vi "Project_GUI.vi"() -> ()   [LabVIEW 2026]
uses:
  <vilib>/Instr/_visa.llb/VISA Configure Serial Port (Instr).vi
panel:
  in  "Display ON/OFF":bool
  in  "stop":bool
  out "Last Command Sent":string
  out "ESP Response":string
  in  "Send Filters":bool
  in  "Detection Threshold":dbl(knob) scale=0.0..255.0
  in  "Blur":dbl(knob) scale=0.0..10.0
  in  "Minimum Area":dbl
  in  "Get Status":bool
  in  "Reset Filters":bool
  in  "Identify":bool
  out "Connected to ESP":bool
  in  "VISA resource name":refnum<visa-resource-name>
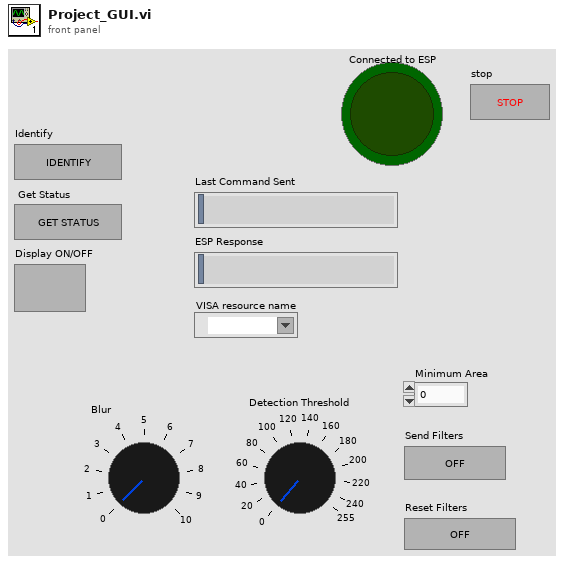
[diagram p1: front panel]
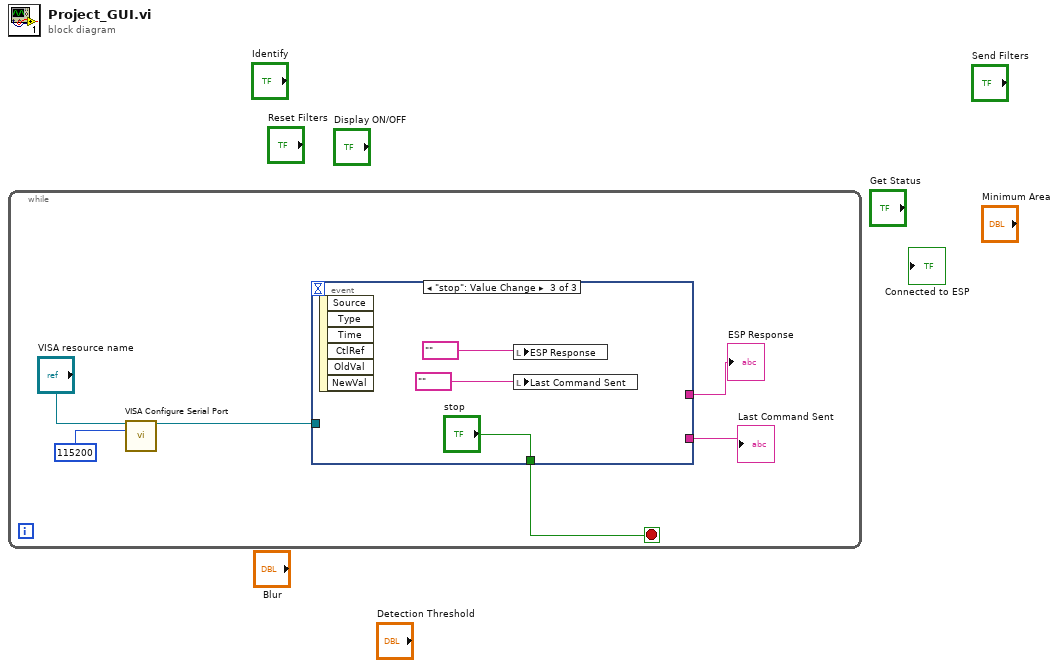
[diagram p0: block diagram]
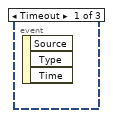
[diagram p2: hidden frame]
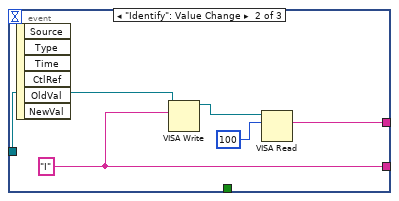
[diagram p3: hidden frame]
diagram:
  n1 = while {
    stop <- w3 stop-if-true
    n2 = call-poly "VISA Configure Serial Port"("VISA resource name"="VISA resource name", "baud rate (9600)"=u32 115200) -> ("VISA resource name out"=w4:refnum<visa-resource-name>)  [unwired: 12 in, 1 out]
    n3 = event shown="[2] \"stop\": Value Change" {
      selector: _ -> [_ _ _]
      dyn-events: _ -> [_ _ _]
      timeout: _ -> [_ _ _]
      tunnel: w4 -> [_ w11 _]
      tunnel: [_ w8 _] -> w2
      tunnel: [_ w7 _] -> w1
      tunnel: [_ _ "stop"] -> w3
      event Timeout {
        n4 = event-data() -> ()  [unwired: 1 in, 3 out]
      }
      event "Identify": Value Change {
        w7 = "I"
        n5 = event-data() -> ()  [unwired: 1 in, 6 out]
        n6 = VISA Write(VISA resource name=w11, write buffer=w7) -> (VISA resource name out=w10:refnum<visa-resource-name>)  [unwired: 1 in, 2 out]
        n7 = VISA Read(VISA resource name=w10, byte count=u32 100) -> (read buffer=w8:string)  [unwired: 1 in, 3 out]
      }
      event "stop": Value Change {
        n8 = event-data() -> ()  [unwired: 1 in, 6 out]
        n9 = local write "ESP Response"("") -> ()
        n10 = local write "Last Command Sent"("") -> ()
      }
    }
    "ESP Response" <- w2
    "Last Command Sent" <- w1
  }
